vi "ReadOpenMVImage.vi"(8 "error in":errorcluster, 11 "VISA Refnum in":refnum<visa-resource-name>) -> (0 "error out":errorcluster, 1 "Good?":bool, 2 "size()":u32[](array[numeric]), 3 "VISA Refnum out":refnum<visa-resource-name>, 4 "image data":T1, 5 "new picture":picture)   [LabVIEW 2016]
uses:
  <vilib>/picture/picture.llb/imagedata.ctl
panel:
  out "read buffer":string
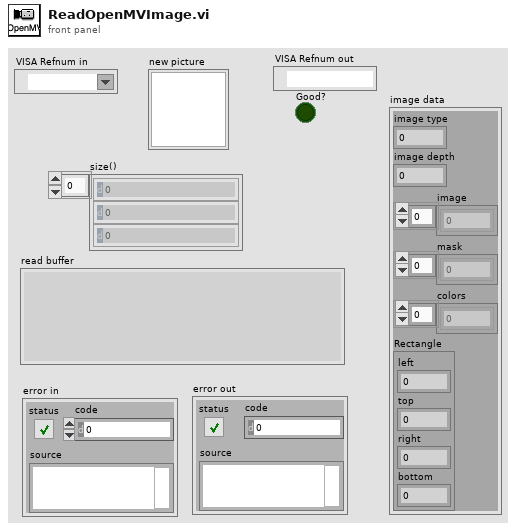
[diagram p1: front panel]
types:
  T1 = typedef "imagedata.ctl" = cluster{"image type":i32, "image depth":i32, "image":u8[], "mask":u8[], "colors":u32[], "Rectangle":cluster{"left":i16, "top":i16, "right":i16, "bottom":i16}}
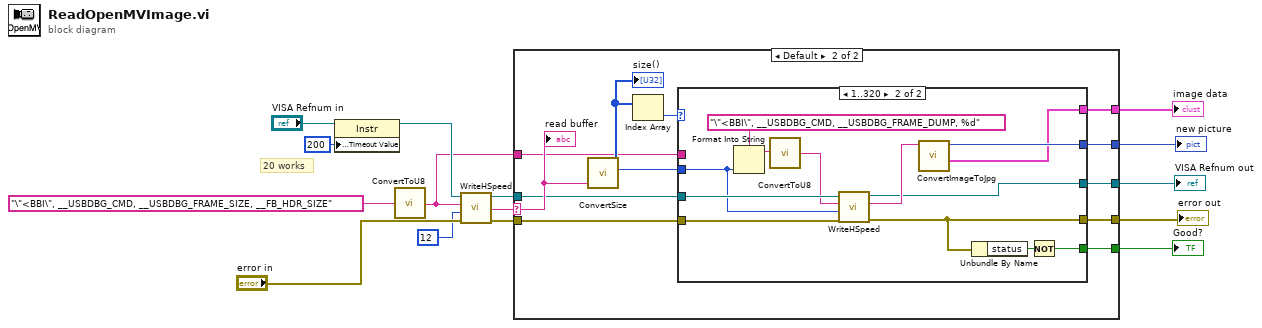
[diagram p0: block diagram]
diagram:
  # "20 works"
  n1 = property class="Instr"(reference="VISA Refnum in", "General Settings:Timeout Value"=u32 200) -> (reference out=w8:refnum<visa-resource-name>)  [unwired: 1 in, 1 out]
  n2 = call "ConvertToU8.vi"("struct"="\"<BBI\", __USBDBG_CMD, __USBDBG_FRAME_SIZE, __FB_HDR_SIZE" ("write buffer")) -> ("Binary"=w1:string)
  n3 = call "WriteHSpeed.vi"("error in"="error in", "Reply length"=12, "write buffer"=w1, "VISA Refnum in"=w8) -> ("error out"=w4:errorcluster, "read buffer"=w3:string, "VISA Refnum out"=w5:refnum<visa-resource-name>)  [unwired: 5 in]
  n4 = case shown="Default" w3 {
    selector: w3 -> [_ w21]
    tunnel: [w17 w29] -> w15
    tunnel: [w16 w28] -> w6
    tunnel: w5 -> [w17 w19]
    tunnel: w4 -> [w16 w25]
    tunnel: [_ w24] -> w13
    tunnel: [_ w23] -> w12
    tunnel: [_ w22] -> w11
    tunnel: w1 -> [_ w18]
    frame "" {
    }
    frame Default {
      n5 = call "ConvertSize.vi"("read buffer"=w21) -> ("# bytes"=w27:u32, "size()"=w20:u32[])  [unwired: 9 in]
      "size()" <- w20
      n6 = Index Array(array=w20) -> (element=w26:u32)  [unwired: 1 in]
      n7 = case shown="1..320" w26 {
        tunnel: [w30 w42] -> w29
        tunnel: [w31 w34] -> w28
        tunnel: w27 -> [_ w40]
        tunnel: w19 -> [w30 w43]
        tunnel: w25 -> [w31 w41]
        tunnel: [_ w36] -> w24
        tunnel: [_ w35] -> w23
        tunnel: [_ w32] -> w22
        tunnel: w18 -> [_ _]
        frame Default {
        }
        frame 1..320 {
          n8 = Format Into String(format string="\"<BBI\", __USBDBG_CMD, __USBDBG_FRAME_DUMP, %d" ("write buffer"), w40) -> (resulting string=w38:string)  [unwired: 2 in, 1 out]
          n9 = call "ConvertToU8.vi"("struct"=w38) -> ("Binary"=w37:string)
          n10 = call "WriteHSpeed.vi"("error in"=w41, "Reply length"=w40, "write buffer"=w37, "VISA Refnum in"=w43) -> ("error out"=w34:errorcluster, "read buffer"=w44:string, "VISA Refnum out"=w42:refnum<visa-resource-name>)  [unwired: 5 in]
          n11 = call "ConvertImageToJpg.vi"("buffer"=w44) -> ("image data"=w35:T1, "new picture"=w36:picture)  [unwired: 9 in]
          n12 = Unbundle By Name(w34) -> ("status"=w33:bool)
          n13 = Not(x=w33) -> (.not. x?=w32:bool)
        }
      }
      "read buffer" <- w21
    }
  }
  "VISA Refnum out" <- w15
  "error out" <- w6
  "new picture" <- w13
  "image data" <- w12
  "Good?" <- w11
